vi "设备名称过滤.vi"(7 "前缀":string, 11 "字符串 i":string="1234f将6") -> (3 "字符串 o":string)   [LabVIEW 2017]
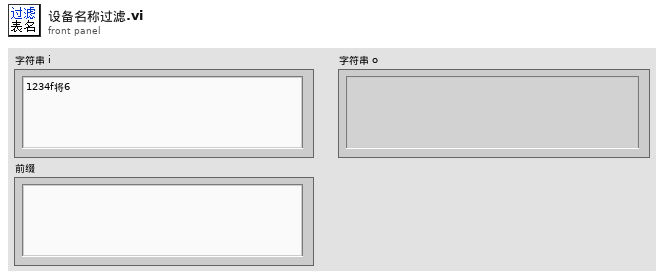
[diagram p1: front panel]
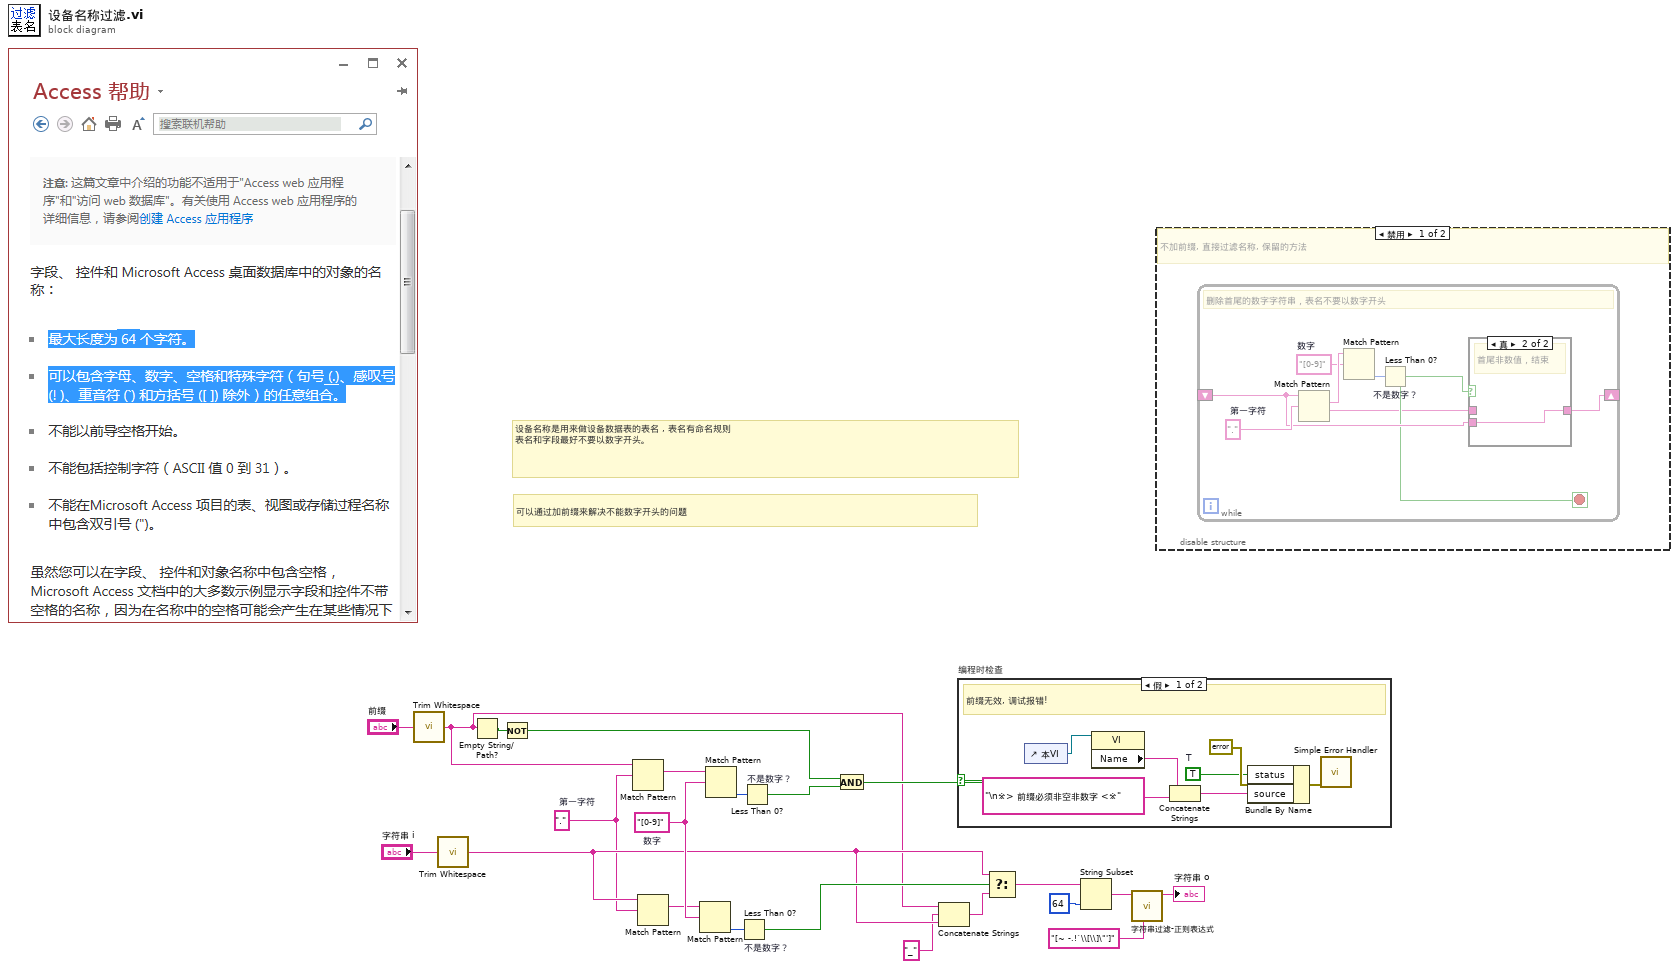
[diagram p0: block diagram]
diagram:
  w6 = "[0-9]"  # 数字
  w4 = "."  # 第一字符
  # "可以通过加前缀来解决不能数字开头的问题"
  # "设备名称是用来做设备数据表的表名 , 表名有命名规则\n表名和字段最好不要以数字开头。"
  n1 = call <vilib>:"Trim Whitespace.vi"("string"="前缀") -> ("trimmed string"=w2:string)  [unwired: 1 in]
  n2 = call <vilib>:"Trim Whitespace.vi"("string"="字符串 i") -> ("trimmed string"=w5:string)  [unwired: 1 in]
  n3 = Empty String/Path?(string/path=w2) -> (empty?=w13:bool)
  n4 = Not(x=w13) -> (.not. x?=w14:bool)
  n5 = Match Pattern(string=w2, regular expression=w4) -> (match substring=w16:string)  [unwired: 1 in, 3 out]
  n6 = Match Pattern(string=w5, regular expression=w4) -> (match substring=w3:string)  [unwired: 1 in, 3 out]
  n7 = Match Pattern(string=w3, regular expression=w6) -> (offset past match=w11:i32)  [unwired: 1 in, 3 out]
  n8 = Match Pattern(string=w16, regular expression=w6) -> (offset past match=w17:i32)  [unwired: 1 in, 3 out]
  n9 = Less Than 0? "不是数字？"(x=w11) -> (x < 0?=w10:bool)
  n10 = Less Than 0? "不是数字？"(x=w17) -> (x < 0?=w7:bool)
  n11 = And(x=w14, y=w7) -> (x .and. y?=w12:bool)
  n12 = Concatenate Strings(w2, "_", w5) -> (w9:string)
  n13 = case "编程时检查" shown="假" w12 {
    frame False {
      w27 = TRUE  # T
      # "前缀无效, 调试报错!"
      n14 = control-ref of="本VI"() -> (w26:refnum<vi>)
      n15 = property class="VI"(reference=w26) -> ("Name"=w24:string)  [unwired: 1 in, 2 out]
      n16 = Concatenate Strings(w24, "\n※> 前缀必须非空非数字 <※") -> (w23:string)
      n17 = Bundle By Name(cluster=errorcluster {"status"=FALSE, "code"=0, "source"=""} ("error in (no error)"), "status"=w27, "source"=w23) -> (w28:errorcluster)
      n18 = call <vilib>:"Simple Error Handler.vi"("error in (no error)"=w28) -> ()  [unwired: 4 in, 5 out]
    }
    frame True {
      # "前缀有效"
    }
  }
  n19 = Select(t=w5, s=w10, f=w9) -> (s? t:f=w8:string)
  n20 = String Subset(string=w8, length (rest)=64 ("长度（剩余）")) -> (substring=w19:string)  [unwired: 1 in]
  n21 = call "字符串过滤-正则表达式.vi"("正则式（非汉字单字符）"="[~ -.!`\\[\\]\"']", "字符串 i"=w19) -> ("字符串 o"=→"字符串 o":string)  [unwired: 8 in, 1 out]
  n22 = disable-structure shown="禁用" {
    frame Disabled {
      # "不加前缀, 直接过滤名称, 保留的方法"
      n23 = while {
        shift-right: [w32] -> _
        shift-left: _ -> [w33]
        stop <- w31 stop-if-true
        w35 = "[0-9]"  # 数字
        w37 = "."  # 第一字符
        # "删除首尾的数字字符串，表名不要以数字开头"
        n24 = Match Pattern(string=w33, regular expression=w37) -> (match substring=w36:string, after substring=w30:string)  [unwired: 1 in, 2 out]
        n25 = Match Pattern(string=w36, regular expression=w35) -> (offset past match=w34:i32)  [unwired: 1 in, 3 out]
        n26 = Less Than 0? "不是数字？"(x=w34) -> (x < 0?=w31:bool)
        n27 = case shown="真" w31 {
          tunnel: w33 -> [_ w39]
          tunnel: [w38 w39] -> w32
          tunnel: w30 -> [w38 _]
          frame False {
            # "去掉首尾"
          }
          frame True {
            # "首尾非数值，结束"
          }
        }
      }
    }
    frame Enabled {
    }
  }
